vi "RT FIFO Variables - host - networked.vi"() -> ()   [LabVIEW 2017]
doc: "This example uses RT FIFO-enabled shared variables to publish data to remote machines without impacting determinism."
panel:
  in  "Amplitude":dbl(slide)=5.0 scale=0.0..10.0
  in  "Stop":bool
  out "Result Data":dbl(graph)=4.653952006038469
  # "Overview: Uses RT FIFO-enabled shared variables to communicate data between loops of different priorities without impacting determinism.\nRequirements: LabVIEW Real-Time Module\nInstructions:\n1. In Measurement & Automation Explorer, ensure that LabVIEW Real-Time and the Network Variable Engine are installed on your RT target.\n2. From the Project Explorer window, set the IP address of your RT target.\n3. Run RT FIFO Variables - host - networked.vi.\n4. Run RT FIFO Variables - target - networked.vi.\n5. From the RT FIFO Variables - host - networked VI front panel, adjust the Amplitude slider, which will update the Result Data chart. \n6. Click the Stop button."
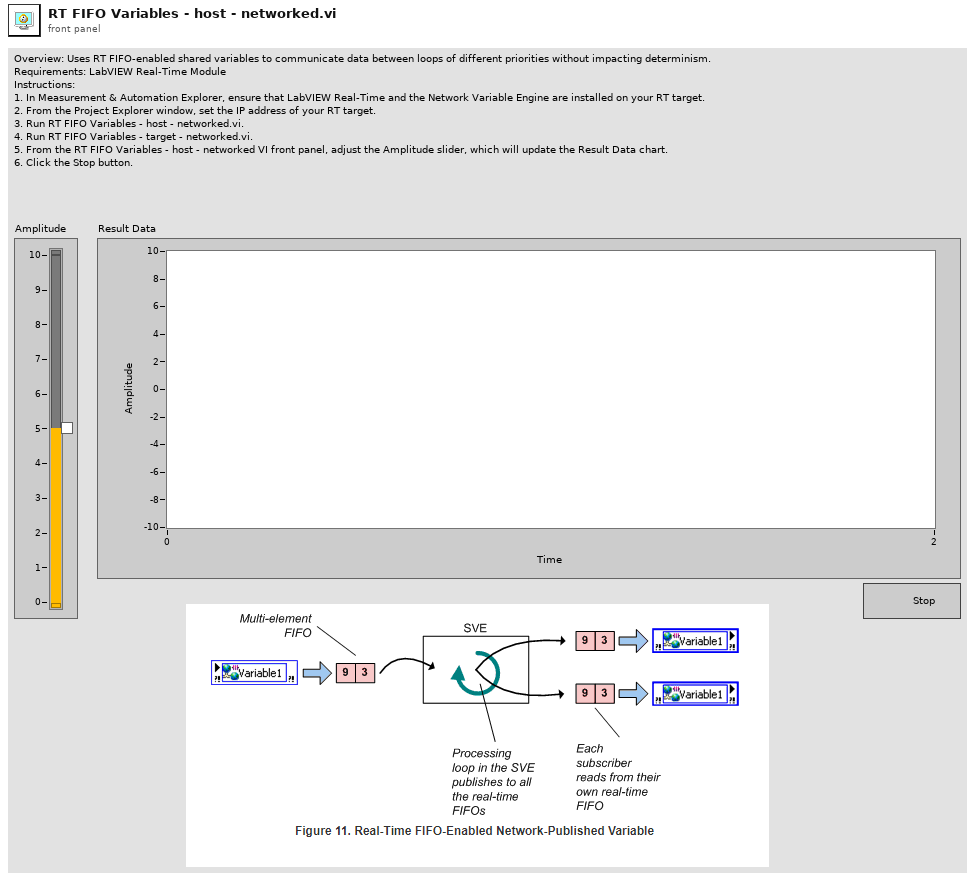
[diagram p1: front panel]
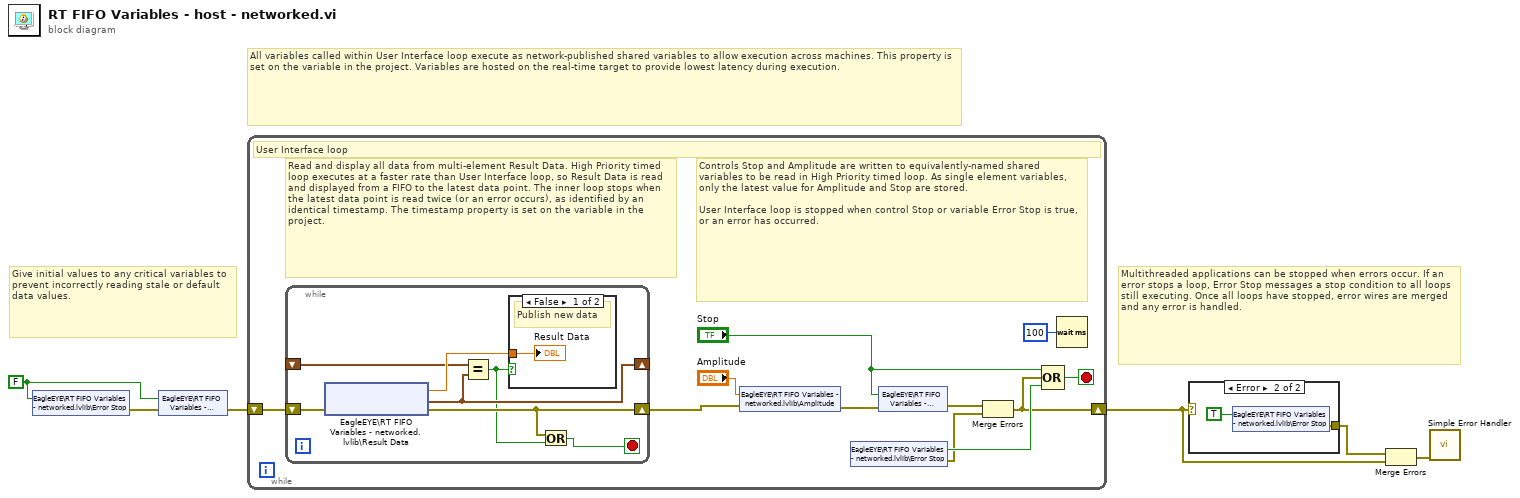
[diagram p0: block diagram]
diagram:
  w4 = FALSE ("Stop")
  # "All variables called within User Interface loop execute as network-published shared variables to allow execution across machines. This property is set on the variable in the project. Variables are hosted on the real-time target to provide lowest latency during execution."
  # "Multithreaded applications can be stopped when errors occur. If an error stops a loop, Error Stop messages a stop condition to all loops still executing. Once all loops have stopped, error wires are merged and any error is handled."
  # "Give initial values to any critical variables to prevent incorrectly reading stale or default data values."
  n1 = shared-variable "EagleEYE\\RT FIFO Variables - networked.lvlib\\Error Stop"(w4) -> (error out=w5:errorcluster)  [unwired: 1 in]
  n2 = shared-variable "EagleEYE\\RT FIFO Variables - networked.lvlib\\Stop"(w4, error in=w5) -> (error out=w6:errorcluster)
  n3 = while "User Interface loop" {
    shift-right: [w8] -> w1
    shift-left: w6 -> [w16]
    stop <- w17 stop-if-true
    # "Controls Stop and Amplitude are written to equivalently-named shared variables to be read in High Priority timed loop. As single element variables, only the latest value for Amplitude and Stop are stored.\n\nUser Interface loop is stopped when control Stop or variable Error Stop is true, or an error has occurred."
    # "Read and display all data from multi-element Result Data. High Priority timed loop executes at a faster rate than User Interface loop, so Result Data is read and displayed from a FIFO to the latest data point. The inner loop stops when the latest data point is read twice (or an error occurs), as identified by an identical timestamp. The timestamp property is set on the variable in the project."
    # "User Interface loop"
    n4 = while {
      shift-right: [w22] -> _
      shift-left: _ -> [w21]
      shift-right: [w20] -> w14
      shift-left: w16 -> [w24]
      stop <- w18 stop-if-true
      n5 = shared-variable "EagleEYE\\RT FIFO Variables - networked.lvlib\\Result Data"(error in=w24) -> (w23:dbl, error out=w20:errorcluster, w22:timestamp)
      n6 = Equal?(x=w21, y=w22) -> (x = y?=w19:bool)
      n7 = case shown="False" w19 {
        tunnel: w23 -> [w25 _]
        frame False {
          # "Publish new data"
          "Result Data" <- w25
        }
        frame True {
          # "No new data"
        }
      }
      n8 = Or(x=w20, y=w19) -> (x .or. y?=w18:bool)
    }
    n9 = shared-variable "EagleEYE\\RT FIFO Variables - networked.lvlib\\Amplitude"("Amplitude", error in=w14) -> (error out=w15:errorcluster)
    n10 = shared-variable "EagleEYE\\RT FIFO Variables - networked.lvlib\\Error Stop"() -> (w10:bool, error out=w7:errorcluster)  [unwired: 1 in]
    n11 = shared-variable "EagleEYE\\RT FIFO Variables - networked.lvlib\\Stop"("Stop", error in=w15) -> (error out=w9:errorcluster)
    n12 = Merge Errors(w9, w7) -> (w8:errorcluster)
    n13 = Compound Arithmetic op=OR("Stop", w8, w10) -> (w17:bool)
    n14 = Wait (ms)(milliseconds to wait=u32 100 ("millisecond multiple")) -> ()  [unwired: 1 out]
  }
  n15 = case shown="Error" w1 {
    tunnel: [_ w26] -> w2
    frame No Error {
    }
    frame Error {
      n16 = shared-variable "EagleEYE\\RT FIFO Variables - networked.lvlib\\Error Stop"(TRUE ("Error Stop")) -> (error out=w26:errorcluster)  [unwired: 1 in]
    }
  }
  n17 = Merge Errors(w2, w1) -> (w3:errorcluster)
  n18 = call <vilib>:"Simple Error Handler.vi"("error in (no error)"=w3) -> ()  [unwired: 4 in, 5 out]
